vi "Set Right.vi"(8 "error in (no error)":errorcluster, 10 "Right":refnum<class "SnailNum.lvclass">, 11 "SnailNum in":refnum<class "SnailNum.lvclass">) -> (0 "error out":errorcluster, 3 "SnailNum out":refnum<class "SnailNum.lvclass">)   [LabVIEW 2020, in "SnailNum.lvclass"]
uses:
  SnailNum.lvclass
  SnailNum.lvclass/SnailNum.ctl
  C:/dev/IlluminatedG/AdventOfCode/2021/source/Day 18/Part 1/SnailElement/SnailElement.lvclass
  C:/dev/IlluminatedG/AdventOfCode/2021/source/Day 18/Part 1/SnailNum/SnailNum.lvclass
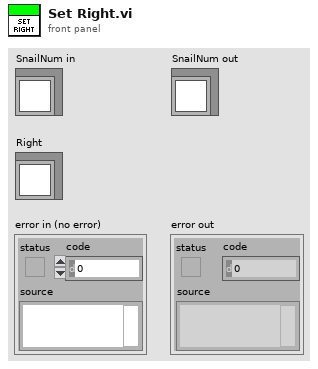
[diagram p1: front panel]
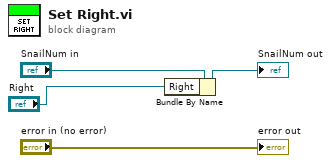
[diagram p0: block diagram]
diagram:
  n1 = Bundle By Name(cluster="SnailNum in", "Right"="Right") -> (→"SnailNum out":refnum<class "SnailNum.lvclass">)
  "error out" <- "error in (no error)"
